vi "UI Main.vi"() -> ()   [LabVIEW 2015]
uses:
  controls/UI Data.ctl
  support/Message Queue/Message Cluster.ctl
  Globals/Global - All UI Loop Stop.vi
  Globals/Global - UI Stream and Variable Connections.vi
  Globals/Global - Configuration Options.vi
  support/User Event - Stop/User Event - Stop.lvlib
  support/Message Queue/Message Queue.lvlib
panel:
  out "Current Logging State":u16(ring) items=["Logging", "Idle (Safe State)"]
  in  "Exit":bool
  out "System Status":string
  in  "Settings Tab":enum32{"UI Commands", "System Monitoring"}(tab)
  in  "Live Data Channel":u32 max=3 step=1
  out "Live Data":waveform(dbl)(graph)
  in  "Stop Live Data":bool
  in  "Acquire Live Data":bool
  out "Most recent manually-triggered log file":path
  in  "Force Trigger":bool
  out "Number of Data Files":u32
  out "Actual Loop Period (ticks)":u32
  out "Largest Contiguous Memory (bytes)":dbl(graph)
  out "Resource Utilization (%)":cluster{dbl, "Double":dbl, dbl}(graph)
  out "System Time":timestamp
  out "Connected?":bool
  in  "Connect to Controller":bool
  in  "Controller Address":string
  # "LabVIEW FPGA Waveform Acquisition and Logging on CompactRIO"
  # "Connection Settings"
  # "Live Data"
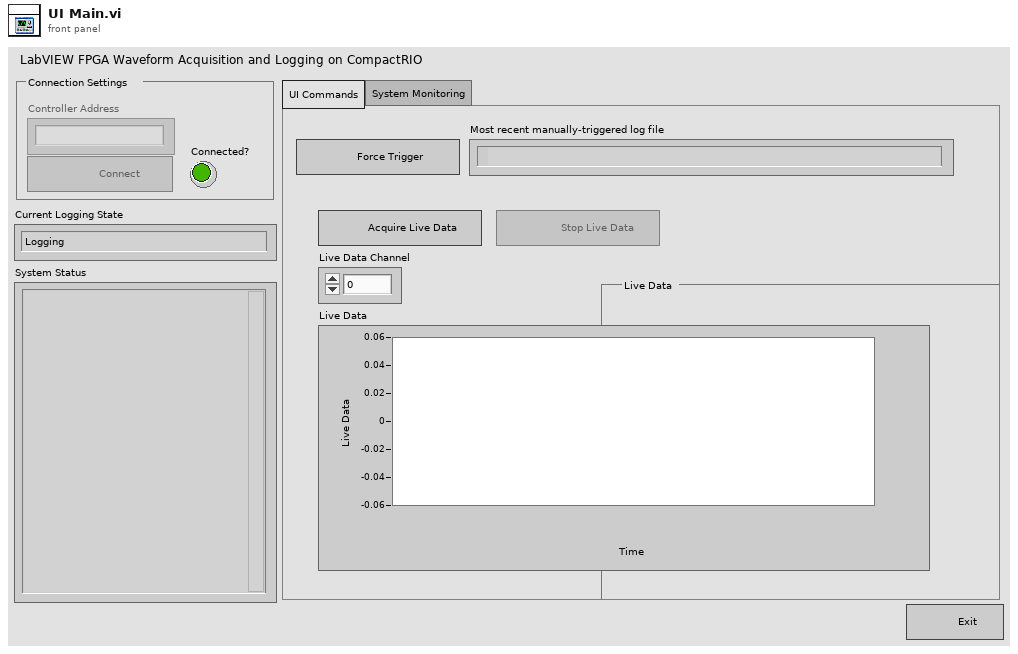
[diagram p1: front panel]
types:
  T1 = typedef "UI Data.ctl" = cluster{"Create Log File Ref":refnum<vi>, "Acquire Live Data Ref":refnum<vi>, "Stop Live Data Ref":refnum<vi>, "Show Live Data Ref":refnum<vi>}
  T2 = typedef "Message Queue.lvlib/All Host Message Queues.ctl" = cluster{"UI":refnum<queue>}
  T3 = typedef "Message Queue.lvlib/Message Cluster.ctl" = cluster{"Message":string, "Message Data":variant}
  T4 = typedef "Variable References.ctl" = cluster{"CPU Usage":refnum<k21>, "Contiguous Memory":refnum<k21>, "Actual Loop Period":refnum<k21>, "Buffer Backlog":refnum<k21>, "Drive Space":refnum<k21>, "Number of Data Files":refnum<k21>, "System Time":refnum<k21>}
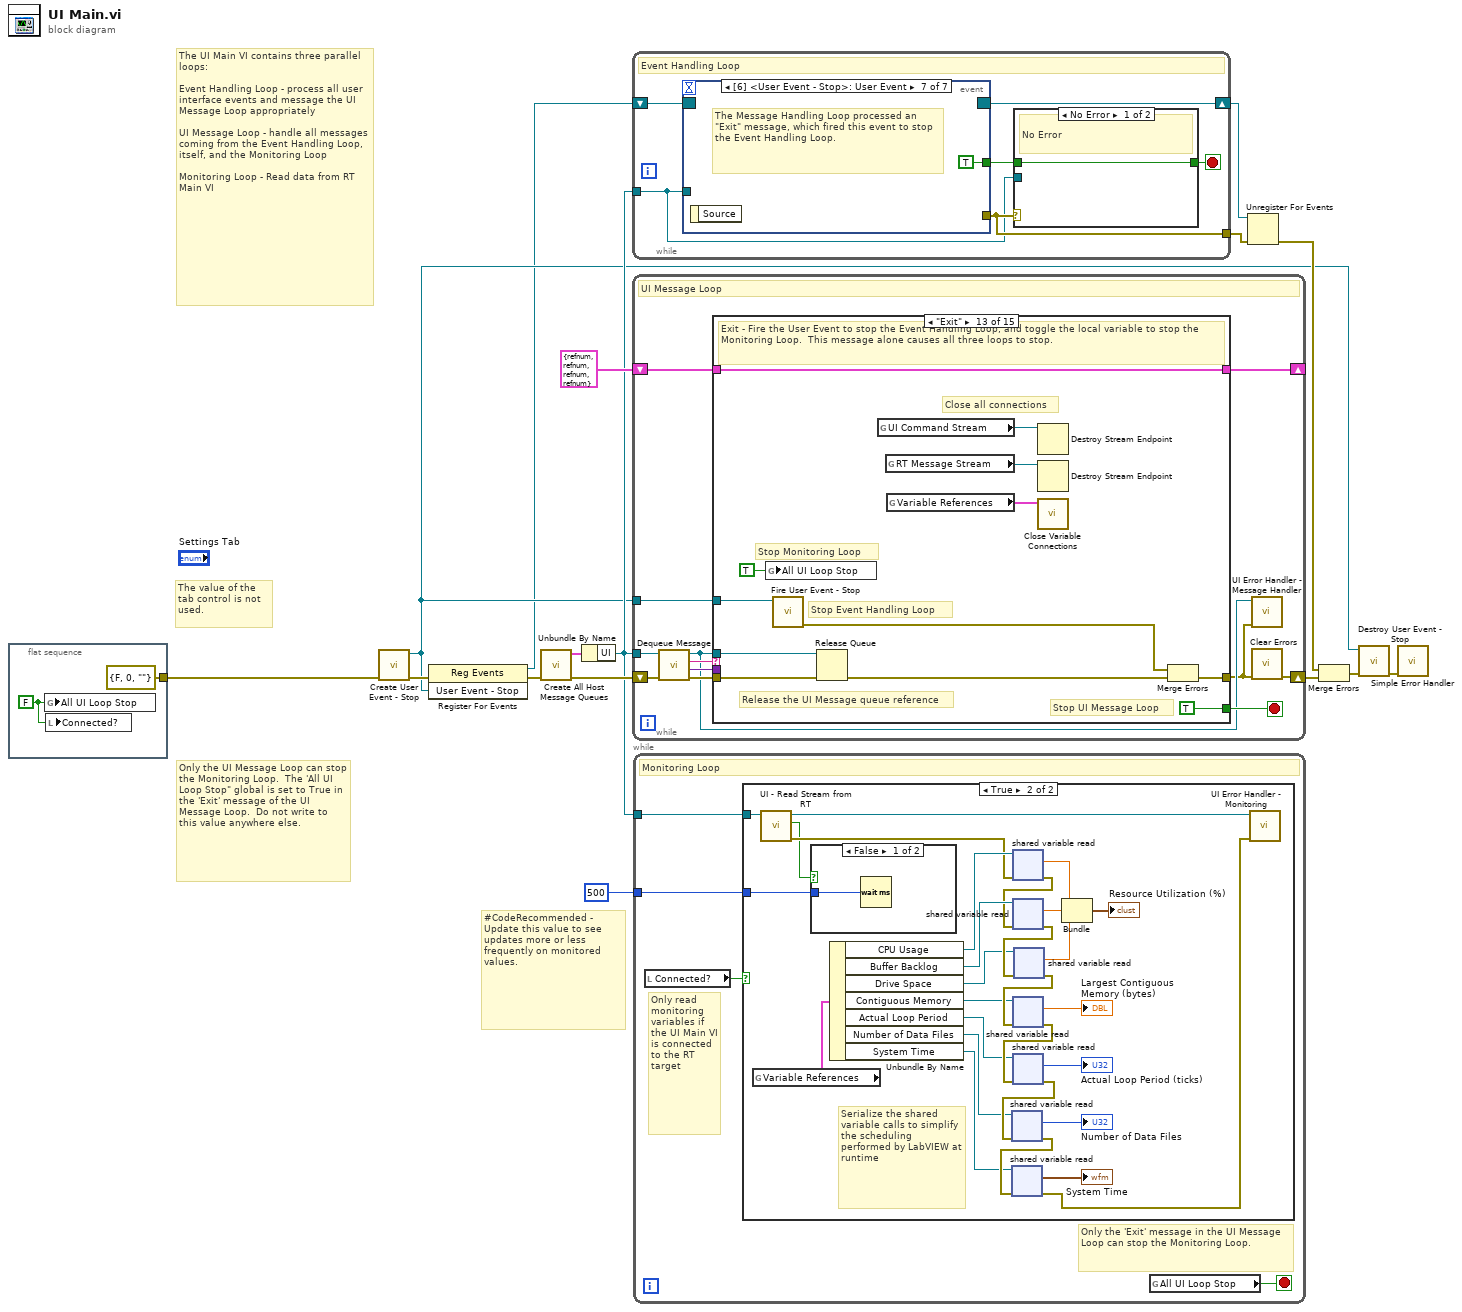
[diagram p0: block diagram]
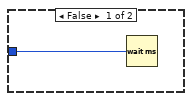
[diagram p2: hidden frame]
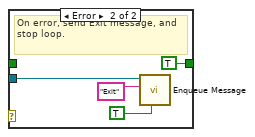
[diagram p4: hidden frame]
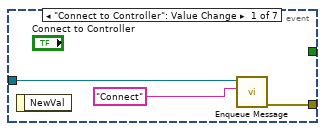
[diagram p5: hidden frame]
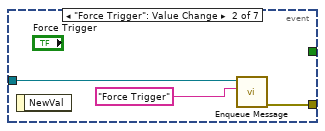
[diagram p6: hidden frame]
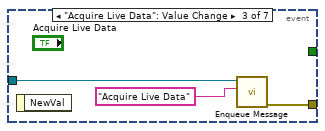
[diagram p7: hidden frame]
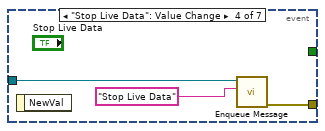
[diagram p8: hidden frame]
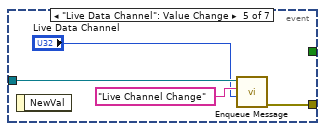
[diagram p9: hidden frame]
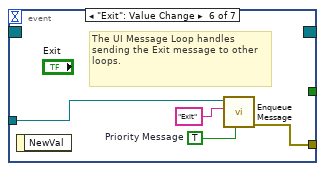
[diagram p10: hidden frame]
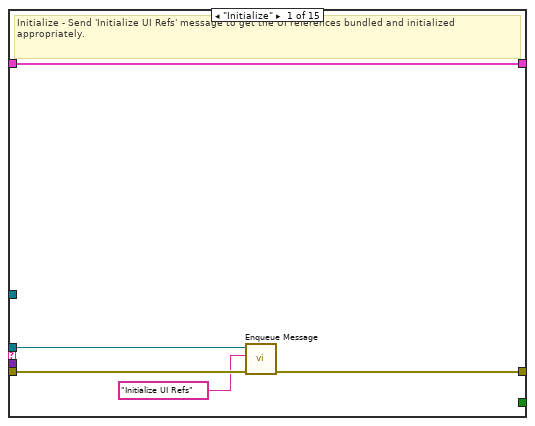
[diagram p11: hidden frame]
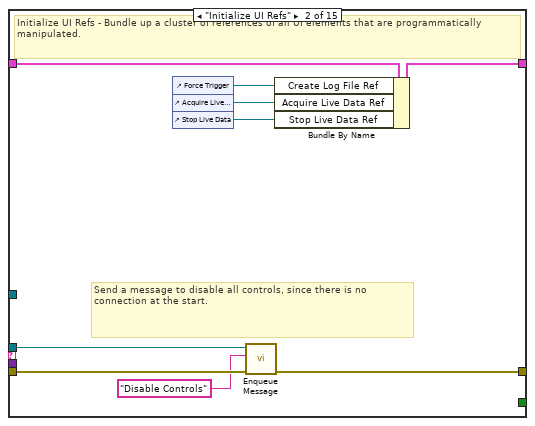
[diagram p12: hidden frame]
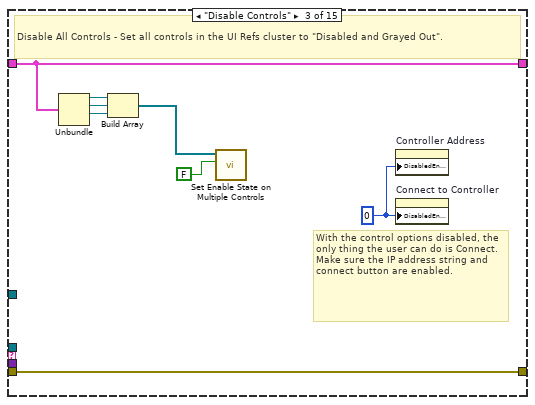
[diagram p13: hidden frame]
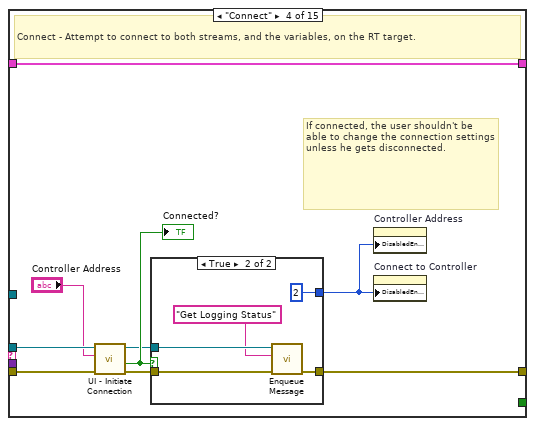
[diagram p14: hidden frame]
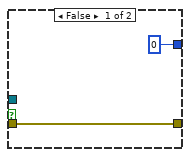
[diagram p15: hidden frame]
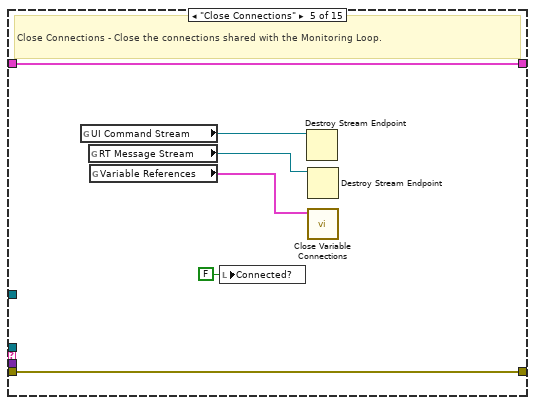
[diagram p16: hidden frame]
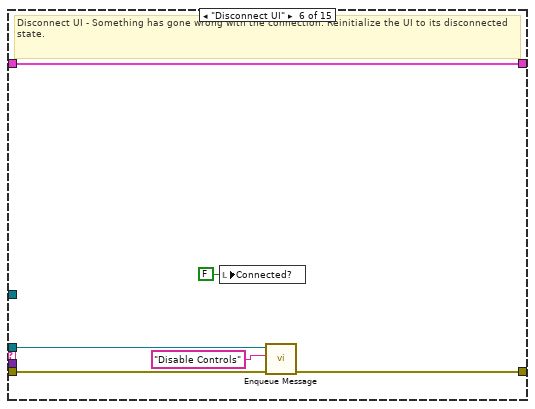
[diagram p17: hidden frame]
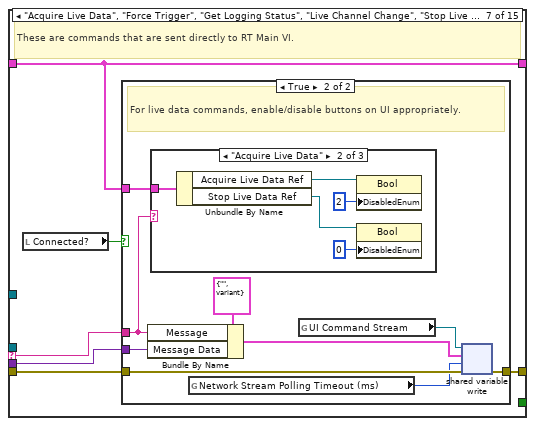
[diagram p18: hidden frame]
diagram:
  # "#CodeRecommended - Update this value to see updates more or less frequently on monitored values."
  # "The UI Main VI contains three parallel loops:\n\nEvent Handling Loop - process all user interface events and message the UI Message Loop appropriately\n\nUI Message Loop - handle all messages coming from the Event Handling Loop, itself, and the Monitoring Loop\n\nMonitoring Loop - Read data from RT Main VI"
  # "The value of the tab control is not used."
  # "Only the UI Message Loop can stop the Monitoring Loop.  The 'All UI Loop Stop\" global is set to True in the 'Exit' message of the UI Message Loop.  Do not write to this value anywhere else."
  n1 = flat-sequence {
    tunnel: [errorcluster {"status"=FALSE, "code"=0, "source"=""} ("error in (no error)")] -> w6
    frame #0 {
      w17 = FALSE
      n2 = global write "Global - All UI Loop Stop.vi" "All UI Loop Stop"(w17) -> ()
      n3 = local write "Connected?"(w17) -> ()
    }
  }
  n4 = call "Create User Event - Stop.vi"("error in (no error)"=w6) -> ("error out"=w4:errorcluster, "User Event - Stop"=w2:refnum<user-event>)  [unwired: 9 in]
  n5 = register-events(error in=w4, w2) -> (reference out=w1:refnum<event-registration>, error out=w3:errorcluster)  [unwired: 1 in]
  n6 = call "Create All Host Message Queues.vi"("error in (no error)"=w3) -> ("error out"=w12:errorcluster, "Message Queues out"=w13:T2)  [unwired: 9 in]
  n7 = Unbundle By Name(w13) -> ("UI"=w7:refnum<queue>)
  n8 = while {
    tunnel: w7 -> [w20]
    tunnel: [w22] -> w15
    shift-right: [w19] -> w10
    shift-left: w1 -> [w21]
    stop <- w23 stop-if-true
    # "Event Handling Loop"
    n9 = event shown="[6] <User Event - Stop>: User Event" {
      selector: w21 -> [_ _ _ _ _ _ _]
      dyn-events: [_ _ _ _ _ _ _] -> w19
      timeout: _ -> [_ _ _ _ _ _ _]
      tunnel: [_ _ _ _ _ _ TRUE ("Discard?")] -> w24
      tunnel: w20 -> [w30 w33 w36 w39 w43 w46 _]
      tunnel: [w32 w35 w38 w41 w45 w49 _] -> w22
      event "Connect to Controller": Value Change {
        n10 = event-data() -> ()  [unwired: 1 in, 1 out]
        n11 = call "Enqueue Message.vi"("Message"="Connect", "Message Queue"=w30) -> ("error out"=w32:errorcluster)  [unwired: 8 in, 1 out]
      }
      event "Force Trigger": Value Change {
        n12 = event-data() -> ()  [unwired: 1 in, 1 out]
        n13 = call "Enqueue Message.vi"("Message"="Force Trigger", "Message Queue"=w33) -> ("error out"=w35:errorcluster)  [unwired: 8 in, 1 out]
      }
      event "Acquire Live Data": Value Change {
        n14 = event-data() -> ()  [unwired: 1 in, 1 out]
        n15 = call "Enqueue Message.vi"("Message"="Acquire Live Data", "Message Queue"=w36) -> ("error out"=w38:errorcluster)  [unwired: 8 in, 1 out]
      }
      event "Stop Live Data": Value Change {
        n16 = event-data() -> ()  [unwired: 1 in, 1 out]
        n17 = call "Enqueue Message.vi"("Message"="Stop Live Data", "Message Queue"=w39) -> ("error out"=w41:errorcluster)  [unwired: 8 in, 1 out]
      }
      event "Live Data Channel": Value Change {
        n18 = event-data() -> ()  [unwired: 1 in, 1 out]
        n19 = call "Enqueue Message.vi"("Message Data"="Live Data Channel", "Message"="Live Channel Change", "Message Queue"=w43) -> ("error out"=w45:errorcluster)  [unwired: 7 in, 1 out]
      }
      event "Exit": Value Change {
        w47 = TRUE  # Priority Message
        # "The UI Message Loop handles sending the Exit message to other loops."
        n20 = event-data() -> ()  [unwired: 1 in, 1 out]
        n21 = call "Enqueue Message.vi"("Priority Message? (F)"=w47, "Message"="Exit", "Message Queue"=w46) -> ("error out"=w49:errorcluster)  [unwired: 7 in, 1 out]
      }
      event User Event {
        # "The Message Handling Loop processed an \"Exit\" message, which fired this event to stop the Event Handling Loop."
        n22 = event-data() -> ()  [unwired: 1 in, 1 out]
      }
    }
    n23 = case shown="No Error" w22 {
      tunnel: [w25 TRUE ("Discard?")] -> w23
      tunnel: w24 -> [w25 _]
      tunnel: w20 -> [_ w26]
      frame No Error {
        # "No Error"
      }
      frame Error {
        # "On error, send Exit message, and stop loop."
        n24 = call "Enqueue Message.vi"("Priority Message? (F)"=TRUE ("Discard?"), "Message"="Exit", "Message Queue"=w26) -> ()  [unwired: 7 in, 2 out]
      }
    }
  }
  n25 = while {
    tunnel: w7 -> [w56]
    tunnel: w2 -> [w61]
    shift-right: [w51] -> w16
    shift-left: w12 -> [w60]
    shift-right: [w54] -> _
    shift-left: T1 {"Create Log File Ref"=refnum, "Acquire Live Data Ref"=refnum, "Stop Live Data Ref"=refnum, "Show Live Data Ref"=refnum} ("Measurement UI Controls") -> [w55]
    stop <- w62 stop-if-true
    # "UI Message Loop"
    n26 = call "Dequeue Message.vi"("error in (no error)"=w60, "Message Queue"=w56) -> ("error out"=w59:errorcluster, "Message Data"=w57:variant, "Message"=w58:string, "dup Message Queue"=w53:refnum<queue>)  [unwired: 6 in]
    n27 = case "Message Cases" shown="\"Exit\"" w58 {
      selector: w58 -> [_ _ _ _ _ _ w115 _ _ _ w167 _ _ _ w228]
      tunnel: w53 -> [w64 w72 _ w92 _ w108 _ _ _ _ w171 _ w213 _ _]
      tunnel: w59 -> [w66 w76 w84 w93 w106 w110 w118 w144 w150 w165 w181 w202 w218 w223 _]
      tunnel: [w65 w73 w84 w87 w106 w109 w117 w142 w148 w164 w182 w200 w219 w222 w226] -> w52
      tunnel: [_ _ _ _ _ _ _ _ _ _ _ _ TRUE _ _] -> w62
      tunnel: w57 -> [_ _ _ _ _ _ w116 w141 w147 w163 w179 w199 _ _ _]
      tunnel: w61 -> [_ _ _ _ _ _ _ _ _ _ _ _ w217 _ _]
      tunnel: w55 -> [w67 w75 w83 w91 w105 w112 w114 w143 w149 w158 w183 w201 w215 w221 w224]
      tunnel: [w67 w74 w83 w91 w105 w112 w114 w143 w149 w158 w183 w201 w215 w221 w224] -> w54
      frame "Initialize" {
        # "Initialize - Send 'Initialize UI Refs' message to get the UI references bundled and initialized appropriately."
        n28 = call "Enqueue Message.vi"("error in (no error)"=w66, "Message"="Initialize UI Refs", "Message Queue"=w64) -> ("error out"=w65:errorcluster)  [unwired: 7 in, 1 out]
      }
      frame "Initialize UI Refs" {
        # "Send a message to disable all controls, since there is no connection at the start."
        # "Initialize UI Refs - Bundle up a cluster of references of all UI elements that are programmatically manipulated."
        n29 = control-ref of="Force Trigger"() -> (w70:refnum<vi>)
        n30 = control-ref of="Acquire Live Data"() -> (w69:refnum<vi>)
        n31 = control-ref of="Stop Live Data"() -> (w68:refnum<vi>)
        n32 = call "Enqueue Message.vi"("error in (no error)"=w76, "Message"="Disable Controls", "Message Queue"=w72) -> ("error out"=w73:errorcluster)  [unwired: 7 in, 1 out]
        n33 = Bundle By Name(cluster=w75, "Create Log File Ref"=w70, "Acquire Live Data Ref"=w69, "Stop Live Data Ref"=w68) -> (w74:T1)
      }
      frame "Disable Controls" {
        w79 = 0
        # "With the control options disabled, the only thing the user can do is Connect. Make sure the IP address string and connect button are enabled."
        # "Disable All Controls - Set all controls in the UI Refs cluster to \"Disabled and Grayed Out\"."
        n34 = Unbundle(w83) -> ("Create Log File Ref"=w82:refnum<vi>, "Acquire Live Data Ref"=w78:refnum<vi>, "Stop Live Data Ref"=w77:refnum<vi>)  [unwired: 1 out]
        n35 = Build Array(w82, w78, w77) -> (w81:refnum<vi>[])
        n36 = call "Set Enable State on Multiple Controls.vi"("Enable?"=FALSE, "Controls"=w81) -> ()  [unwired: 10 in]
        n37 = property on="Controller Address" class="Str"("DisabledEnum"=w79) -> ()  [unwired: 2 in, 2 out]
        n38 = property on="Connect to Controller" class="Bool"("DisabledEnum"=w79) -> ()  [unwired: 2 in, 2 out]
      }
      frame "Connect" {
        # "If connected, the user shouldn't be able to change the connection settings unless he gets disconnected."
        # "Connect - Attempt to connect to both streams, and the variables, on the RT target."
        n39 = call "UI - Initiate Connection.vi"("error in (no error)"=w93, "Controller Address"="Controller Address", "Message Queue"=w92) -> ("error out"=w89:errorcluster, "Connected?"=w88:bool, "dup Message Queue"=w86:refnum<queue>)  [unwired: 6 in]
        "Connected?" <- w88
        n40 = case shown="True" w88 {
          tunnel: w89 -> [w95 w99]
          tunnel: [w95 w100] -> w87
          tunnel: w86 -> [_ w98]
          tunnel: [0 2] -> w85
          frame False {
          }
          frame True {
            n41 = call "Enqueue Message.vi"("error in (no error)"=w99, "Message"="Get Logging Status", "Message Queue"=w98) -> ("error out"=w100:errorcluster)  [unwired: 7 in, 1 out]
          }
        }
        n42 = property on="Controller Address" class="Str"("DisabledEnum"=w85) -> ()  [unwired: 2 in, 2 out]
        n43 = property on="Connect to Controller" class="Bool"("DisabledEnum"=w85) -> ()  [unwired: 2 in, 2 out]
      }
      frame "Close Connections" {
        # "Close Connections - Close the connections shared with the Monitoring Loop."
        n44 = global read "Global - UI Stream and Variable Connections.vi" "UI Command Stream"() -> (w104:refnum<k21>)
        n45 = global read "Global - UI Stream and Variable Connections.vi" "RT Message Stream"() -> (w103:refnum<k21>)
        n46 = global read "Global - UI Stream and Variable Connections.vi" "Variable References"() -> (w102:T4)
        n47 = local write "Connected?"(FALSE ("Connected?")) -> ()
        n48 = Destroy Stream Endpoint(11:w104) -> ()  [unwired: 1 in, 1 out]
        n49 = Destroy Stream Endpoint(11:w103) -> ()  [unwired: 1 in, 1 out]
        n50 = call "Close Variable Connections.vi"("Variable References"=w102) -> ()  [unwired: 11 in]
      }
      frame "Disconnect UI" {
        # "Disconnect UI - Something has gone wrong with the connection. Reinitialize the UI to its disconnected state."
        n51 = local write "Connected?"(FALSE ("Connected?")) -> ()
        n52 = call "Enqueue Message.vi"("error in (no error)"=w110, "Message"="Disable Controls", "Message Queue"=w108) -> ("error out"=w109:errorcluster)  [unwired: 7 in, 1 out]
      }
      frame "Acquire Live Data", "Force Trigger", "Get Logging Status", "Live Channel Change", "Stop Live Data" {
        # "These are commands that are sent directly to RT Main VI."
        n53 = local read "Connected?"() -> (w113:bool)
        n54 = case shown="True" w113 {
          tunnel: w118 -> [w119 w128]
          tunnel: [w119 w127] -> w117
          tunnel: w116 -> [_ w122]
          tunnel: w115 -> [_ w120]
          tunnel: w114 -> [_ w121]
          frame False {
            # "Don't bother trying to send a message to the RT system if UI Main VI isn't even connected"
          }
          frame True {
            # "For live data commands, enable/disable buttons on UI appropriately."
            n55 = Bundle By Name(cluster=T3 {"Message"="", "Message Data"=variant} ("Message Cluster"), "Message"=w120, "Message Data"=w122) -> (w123:T3)
            n56 = case shown="\"Acquire Live Data\"" w120 {
              tunnel: w121 -> [_ w133 w138]
              frame Default {
              }
              frame "Acquire Live Data" {
                n57 = Unbundle By Name(w133) -> ("Acquire Live Data Ref"=w132:refnum<vi>, "Stop Live Data Ref"=w131:refnum<vi>)
                n58 = property class="Bool"(reference=w132, "DisabledEnum"=u8 2) -> ()  [unwired: 1 in, 2 out]
                n59 = property class="Bool"(reference=w131, "DisabledEnum"=u8 0) -> ()  [unwired: 1 in, 2 out]
              }
              frame "Stop Live Data" {
                n60 = Unbundle By Name(w138) -> ("Acquire Live Data Ref"=w137:refnum<vi>, "Stop Live Data Ref"=w136:refnum<vi>)
                n61 = property class="Bool"(reference=w137, "DisabledEnum"=u8 0) -> ()  [unwired: 1 in, 2 out]
                n62 = property class="Bool"(reference=w136, "DisabledEnum"=u8 2) -> ()  [unwired: 1 in, 2 out]
              }
            }
            n63 = global read "Global - Configuration Options.vi" "Network Stream Polling Timeout (ms)"() -> (w125:i32)
            n64 = global read "Global - UI Stream and Variable Connections.vi" "UI Command Stream"() -> (w126:refnum<k21>)
            n65 = shared-variable-write(w126, w128, w123, w125) -> (w127:errorcluster)  [unwired: 2 out]
          }
        }
      }
      frame "Send Path to UI" {
        # "Send Path to UI - Message from the RT Main VI containing the path to the manually-triggered log file."
        n66 = Variant To Data(error in=w144, type=path "", Variant=w141) -> (data=→"Most recent manually-triggered log file":path, error out=w142:errorcluster)
      }
      frame "Send Live Data to UI" {
        # "Send Live Data to UI - Message from the RT Main VI containing the latest live data for the specified channel."
        n67 = Variant To Data(error in=w150, type=waveform(dbl) {"t0"=timestamp(0 s since 1904-01-01), "dt"=1.0, "Y"=[]}, Variant=w147) -> (data=→"Live Data":waveform(dbl), error out=w148:errorcluster)
      }
      frame "Send Logging Status" {
        # "TRUE: Logging Normally\nFALSE: Idle (Safe State)"
        # "Send Logging Status - Message from the RT Main VI indicating whether or not logging is happening normally, or if the logging loop is in safe mode."
        n68 = Unbundle By Name(w158) -> ("Create Log File Ref"=w157:refnum<vi>, "Acquire Live Data Ref"=w156:refnum<vi>, "Stop Live Data Ref"=w152:refnum<vi>)
        n69 = Variant To Data(error in=w165, type=FALSE, Variant=w163) -> (data=w153:bool, error out=w164:errorcluster)
        n70 = Build Array(w157, w156) -> (w155:refnum<vi>[])
        n71 = Build Array(w152) -> (w154:refnum<vi>[])
        n72 = Select(t=u16 0, s=w153, f=u16 1) -> (s? t:f=→"Current Logging State":u16)
        n73 = call "Set Enable State on Multiple Controls.vi"("Enable?"=w153, "Controls"=w155) -> ()  [unwired: 10 in]
        n74 = call "Set Enable State on Multiple Controls.vi"("Enable?"=FALSE, "Controls"=w154) -> ()  [unwired: 10 in]
      }
      frame "Critical Error", "Log-Only Error", "Non-Critical Error", "RT Error" {
        # "Error - Display message in status indicator on panel.  If it's a critical error, shut down this VI with an 'Exit' message."
        n75 = case shown="Default" w167 {
          selector: w167 -> [_ w185]
          tunnel: ["UI Error" w185] -> w166
          frame Default {
          }
          frame "RT Error" {
          }
        }
        n76 = Variant To Data(error in=w181, type=errorcluster {"status"=FALSE, "code"=0, "source"=""} ("error constant"), Variant=w179) -> (data=w174:errorcluster, error out=w180:errorcluster)
        n77 = Unbundle By Name(w174) -> ("code"=w173:i32, "source"=w177:string)
        n78 = Format Date/Time String() -> (date/time string=w176:string)  [unwired: 3 in]
        n79 = Format Into String(format string="\n%s: %s %d - %s", w176, w166, w173, w177) -> (resulting string=w168:string)  [unwired: 2 in, 1 out]
        n80 = call "Enqueue Message.vi"("error in (no error)"=w180, "Message Data"=w168, "Message"="Update System Status", "Message Queue"=w171) -> ("error out"=w172:errorcluster, "dup Message Queue"=w170:refnum<queue>)  [unwired: 6 in]
        n81 = case shown="Default" w167 {
          tunnel: w172 -> [w186 w190]
          tunnel: w170 -> [_ w188]
          tunnel: [w186 w189] -> w182
          frame Default {
          }
          frame "Critical Error" {
            n82 = call "Enqueue Message.vi"("error in (no error)"=w190, "Message"="Exit", "Message Queue"=w188) -> ("error out"=w189:errorcluster)  [unwired: 7 in, 1 out]
          }
        }
      }
      frame "Update System Status" {
        # "#CodeRecommended - The code below ensures that the System Status string value does not become too large.  It uses the same maximum size as the RT error log to determine whether or not to remove the last half of the log string. Change this logic if you wish to maintain more/less of the information in the System Status string."
        # "Update System Status - Add a new string to the beginning of the System Status string on the UI."
        n83 = Variant To Data(error in=w202, type="", Variant=w199) -> (data=w196:string, error out=w200:errorcluster)
        n84 = global read "Global - Configuration Options.vi" "Error Log Max Size (bytes)"() -> (w192:i64)
        n85 = local read "System Status"() -> (w194:string)
        n86 = String Length(string=w194) -> (length=w195:i32)
        n87 = Greater?(x=w195, y=w192) -> (0:w193:bool)
        n88 = case shown="True" w193 {
          tunnel: w194 -> [w203 w207]
          tunnel: w192 -> [_ w206]
          tunnel: [w203 w208] -> w191
          frame False {
          }
          frame True {
            n89 = Divide(x=w206, y=i64 2) -> (x/y=w205:dbl)
            n90 = String Subset(string=w207, length (rest)=w205) -> (substring=w208:string)  [unwired: 1 in]
          }
        }
        n91 = Concatenate Strings(w196, w191) -> (→"System Status":string)
      }
      frame "Exit" {
        # "Close all connections"
        # "Stop Monitoring Loop"
        # "Stop Event Handling Loop"
        # "Release the UI Message queue reference"
        # "Stop UI Message Loop"
        # "Exit - Fire the User Event to stop the Event Handling Loop, and toggle the local variable to stop the Monitoring Loop.  This message alone causes all three loops to stop."
        n92 = global write "Global - All UI Loop Stop.vi" "All UI Loop Stop"(TRUE ("Stop Monitoring Loop")) -> ()
        n93 = call "Fire User Event - Stop.vi"("User Event - Stop"=w217) -> ("error out"=w216:errorcluster)  [unwired: 10 in]
        n94 = Release Queue(queue=w213, error in (no error)=w218) -> (error out=w214:errorcluster)  [unwired: 1 in, 2 out]
        n95 = global read "Global - UI Stream and Variable Connections.vi" "UI Command Stream"() -> (w211:refnum<k21>)
        n96 = global read "Global - UI Stream and Variable Connections.vi" "RT Message Stream"() -> (w210:refnum<k21>)
        n97 = global read "Global - UI Stream and Variable Connections.vi" "Variable References"() -> (w209:T4)
        n98 = Destroy Stream Endpoint(11:w211) -> ()  [unwired: 1 in, 1 out]
        n99 = Destroy Stream Endpoint(11:w210) -> ()  [unwired: 1 in, 1 out]
        n100 = call "Close Variable Connections.vi"("Variable References"=w209) -> ()  [unwired: 11 in]
        n101 = Merge Errors(w216, w214) -> (w219:errorcluster)
      }
      frame "---Copy This Frame---" {
        # "Duplicate this frame when creating new messages.  Change this comment in the duplicated frame to describe this message."
        n102 = Merge Errors(w223) -> (w222:errorcluster)
      }
      frame Default {
        # "'Default' case only runs if there is a message that isn't defined in any of the other cases.  Output a programming error."
        n103 = Format Into String(format string="The invalid message string \"%s\" was received in the Message Handling Loop." ("Invalid Message Loop Message"), w228) -> (resulting string=w225:string)  [unwired: 2 in, 1 out]
        n104 = call <vilib>:"Error Cluster From Error Code.vi"("error message (\"\")"=w225, "error code (0)"=1) -> ("error out"=w226:errorcluster)  [unwired: 7 in]
      }
    }
    n105 = call "UI Error Handler - Message Handler.vi"("error in (no error)"=w52, "Message Queue"=w53) -> ()  [unwired: 9 in, 1 out]
    n106 = call <vilib>:"Clear Errors.vi"("error in (no error)"=w52) -> ("error out"=w51:errorcluster)  [unwired: 5 in, 1 out]
  }
  n107 = while {
    tunnel: w7 -> [w232]
    tunnel: u32 500 ("milliseconds to wait") -> [w230]
    stop <- w233 stop-if-true
    # "Only read monitoring variables if the UI Main VI is connected to the RT target"
    # "Only the 'Exit' message in the UI Message Loop can stop the Monitoring Loop."
    # "Monitoring Loop"
    n108 = local read "Connected?"() -> (w231:bool)
    n109 = case shown="True" w231 {
      tunnel: w232 -> [_ w258]
      tunnel: w230 -> [w234 w235]
      frame False {
        n110 = Wait (ms)(milliseconds to wait=w234) -> ()  [unwired: 1 out]
      }
      frame True {
        # "Serialize the shared variable calls to simplify the scheduling performed by LabVIEW at runtime"
        n111 = global read "Global - UI Stream and Variable Connections.vi" "Variable References"() -> (w256:T4)
        n112 = call "UI - Read Stream from RT.vi"("Message Queue"=w258) -> ("error out"=w259:errorcluster, "Message Received?"=w236:bool, "dup Message Queue"=w257:refnum<queue>)  [unwired: 8 in]
        n113 = case shown="False" w236 {
          tunnel: w235 -> [w263 _]
          frame False {
            n114 = Wait (ms)(milliseconds to wait=w263) -> ()  [unwired: 1 out]
          }
          frame True {
            # "If a message was received, immediately read again"
          }
        }
        n115 = Unbundle By Name(w256) -> ("CPU Usage"=w261:refnum<k21>, "Buffer Backlog"=w260:refnum<k21>, "Drive Space"=w237:refnum<k21>, "Contiguous Memory"=w248:refnum<k21>, "Actual Loop Period"=w245:refnum<k21>, "Number of Data Files"=w242:refnum<k21>, "System Time"=w238:refnum<k21>)
        n116 = shared-variable-read(w261, w259) -> (w255:errorcluster, w253:dbl)  [unwired: 2 out]
        n117 = shared-variable-read(w260, w255) -> (w254:errorcluster, w252:dbl)  [unwired: 2 out]
        n118 = shared-variable-read(w237, w254) -> (w249:errorcluster, w251:dbl)  [unwired: 2 out]
        n119 = shared-variable-read(w248, w249) -> (w246:errorcluster, →"Largest Contiguous Memory (bytes)":dbl)  [unwired: 2 out]
        n120 = shared-variable-read(w245, w246) -> (w244:errorcluster, →"Actual Loop Period (ticks)":u32)  [unwired: 2 out]
        n121 = shared-variable-read(w242, w244) -> (w241:errorcluster, →"Number of Data Files":u32)  [unwired: 2 out]
        n122 = shared-variable-read(w238, w241) -> (w239:errorcluster, →"System Time":timestamp)  [unwired: 2 out]
        n123 = Bundle(w253, "Double"=w252, w251) -> (→"Resource Utilization (%)":cluster{dbl, "Double":dbl, dbl})  [unwired: 1 in]
        n124 = call "UI Error Handler - Monitoring.vi"("error in (no error)"=w239, "Message Queue"=w257) -> ()  [unwired: 9 in, 1 out]
      }
    }
    n125 = global read "Global - All UI Loop Stop.vi" "All UI Loop Stop"() -> (w233:bool)
  }
  n126 = Unregister For Events(event registration refnum=w10, error in=w15) -> (error out=w11:errorcluster)
  n127 = Merge Errors(w11, w16) -> (w14:errorcluster)
  n128 = call "Destroy User Event - Stop.vi"("error in (no error)"=w14, "User Event - Stop"=w2) -> ("error out"=w8:errorcluster)  [unwired: 9 in]
  n129 = call <vilib>:"Simple Error Handler.vi"("error in (no error)"=w8) -> ()  [unwired: 4 in, 5 out]
